vi "2 int to real conversion.vi"(9 "reale in":dbl format="%.20g", 10 "MW 15 0 in":i32=7537, 11 "MW 31 16 in":i32=17309) -> (0 "MW 15 0 out":i16=7537, 1 "MW 31 16 out":i16=17309, 2 "reale out":dbl format="%.20g")   [LabVIEW 2019]
panel:
  out "Boolean array":bool[](array[boolean])
  out "exponent":dbl
  out "mantissa":dbl
  out "appended array 2":bool[](array[boolean])
  out "appended array":bool[](array[boolean])
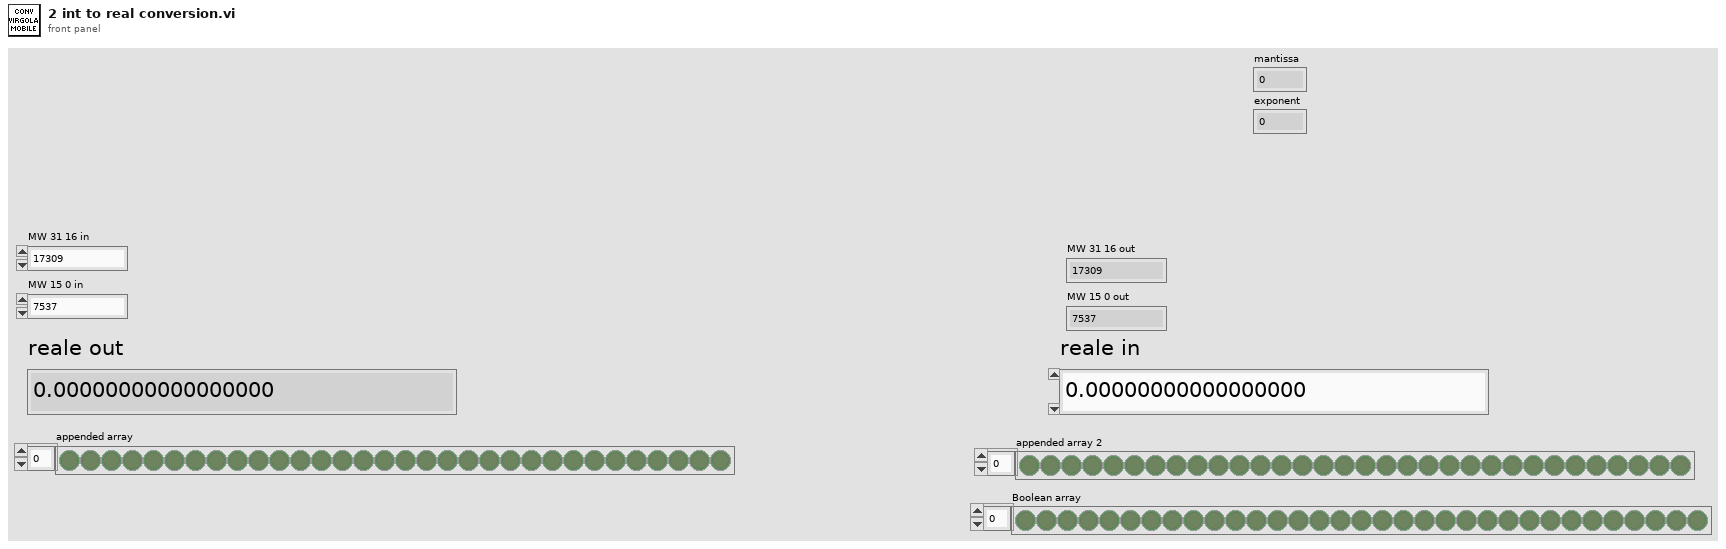
[diagram p1: front panel]
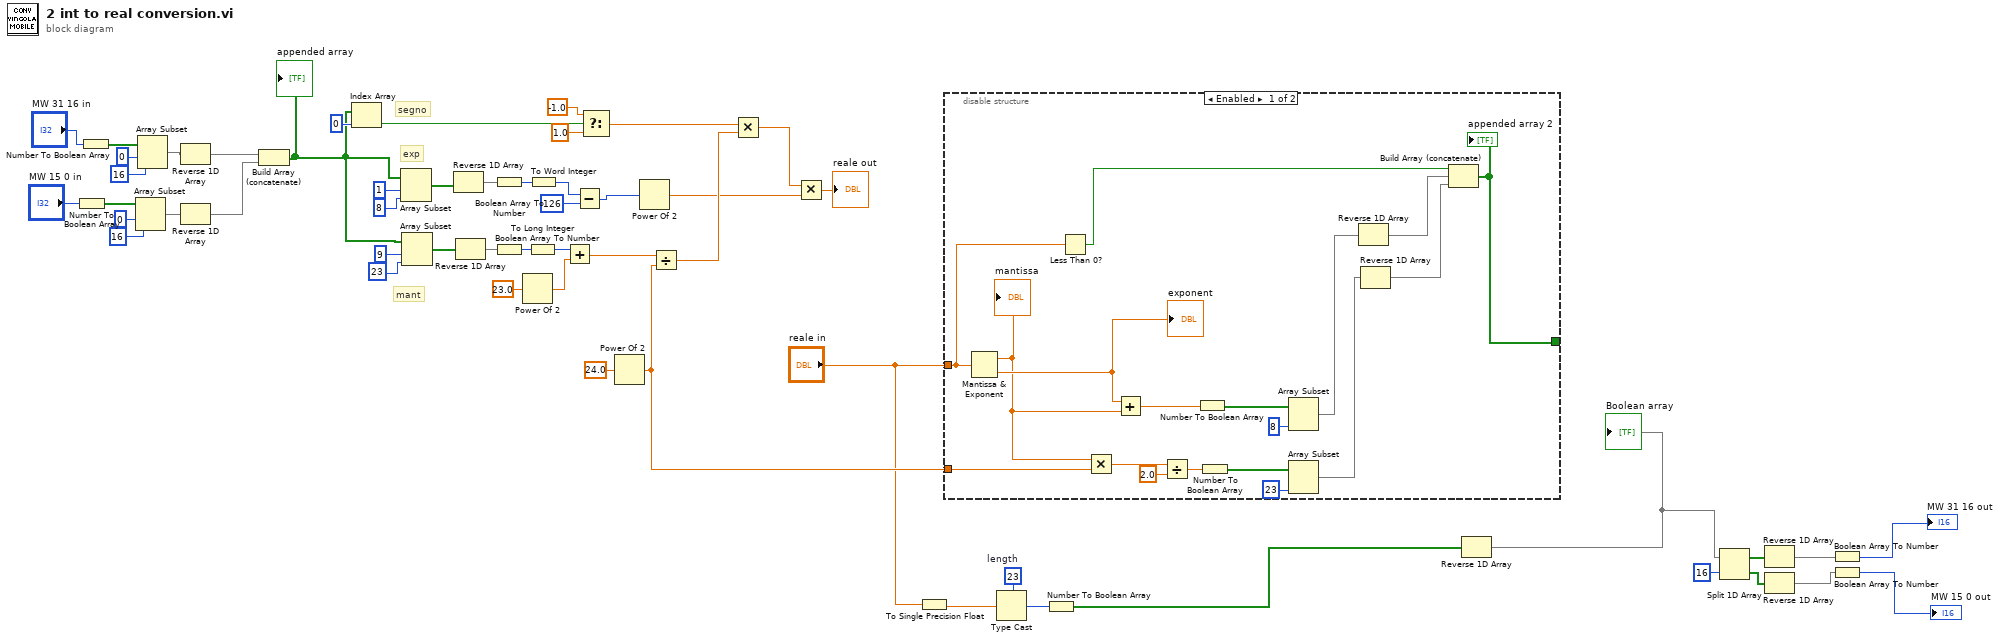
[diagram p0: block diagram]
diagram:
  w8 = 23  # length
  # "mant"
  # "segno"
  # "exp"
  n1 = Number To Boolean Array(number="MW 15 0 in") -> (Boolean array=w54:bool[])
  n2 = Number To Boolean Array(number="MW 31 16 in") -> (Boolean array=w49:bool[])
  n3 = Array Subset(array=w54, index=0, length=16) -> (w35:bool[])
  n4 = Array Subset(array=w49, index=0, length=16) -> (w37:bool[])
  n5 = Reverse 1D Array(array=w37) -> (reversed array=w36:bool[])
  n6 = Reverse 1D Array(array=w35) -> (reversed array=w29:bool[])
  n7 = Build Array (concatenate)(w36, w29) -> (w38:bool[])
  "appended array" <- w38
  n8 = Index Array(array=w38, index=0) -> (element=w33:bool)
  n9 = Array Subset(array=w38, index=1, length=8) -> (w17:bool[])
  n10 = Array Subset(array=w38, index=9, length=23) -> (w18:bool[])
  n11 = Reverse 1D Array(array=w17) -> (reversed array=w16:bool[])
  n12 = Reverse 1D Array(array=w18) -> (reversed array=w15:bool[])
  n13 = Boolean Array To Number(Boolean array=w16) -> (number=w28:u32)
  n14 = Boolean Array To Number(Boolean array=w15) -> (number=w25:u32)
  n15 = Power Of 2(x=23.0) -> (2^x=w12:dbl)
  n16 = To Long Integer(number=w25) -> (32bit integer=w24:i32)
  n17 = To Word Integer(number=w28) -> (16bit integer=w27:i16)
  n18 = Add(x=w24, y=w12) -> (x+y=w39:dbl)
  n19 = Subtract(x=w27, y=i16 126) -> (x-y=w21:i16)
  n20 = Select(t=-1.0 ("y"), s=w33, f=1.0) -> (s? t:f=w32:dbl)
  n21 = Power Of 2(x=24.0) -> (2^x=w11:dbl)
  n22 = Power Of 2(x=w21) -> (2^x=w22:dbl)
  n23 = Divide(x=w39, y=w11) -> (x/y=w23:dbl)
  n24 = Multiply(x=w32, y=w23) -> (x*y=w34:dbl)
  n25 = Multiply(x=w34, y=w22) -> (x*y=→"reale out":dbl)
  n26 = To Single Precision Float(number="reale in") -> (single precision float=w9:sgl)
  n27 = disable-structure shown="Enabled" {
    disable-tunnel: w11 -> [w59 _]
    disable-tunnel: "reale in" -> [w56 _]
    disable-tunnel: [w55 _] -> _
    frame Enabled {
      n28 = Mantissa & Exponent(0:w56) -> (1:w57:dbl, 2:w58:dbl)
      "mantissa" <- w57
      "exponent" <- w58
      n29 = Less Than 0?(x=w56) -> (x < 0?=w71:bool)
      n30 = Multiply(x=w57, y=w59) -> (x*y=w64:dbl)
      n31 = Add(x=w58, y=w57) -> (x+y=w69:dbl)
      n32 = Divide(x=w64, y=2.0) -> (x/y=w65:dbl)
      n33 = Number To Boolean Array(number=w69) -> (Boolean array=w70:bool[])
      n34 = Number To Boolean Array(number=w65) -> (Boolean array=w67:bool[])
      n35 = Array Subset(array=w70, length=8) -> (w63:bool[])  [unwired: 1 in]
      n36 = Array Subset(array=w67, length=23) -> (w62:bool[])  [unwired: 1 in]
      n37 = Reverse 1D Array(array=w63) -> (reversed array=w61:bool[])
      n38 = Reverse 1D Array(array=w62) -> (reversed array=w60:bool[])
      n39 = Build Array (concatenate)(w71, w61, w60) -> (w55:bool[])
      "appended array 2" <- w55
    }
    frame Disabled {
    }
  }
  n40 = Type Cast(type=w8, x=w9) -> (*(type *) &x=w7:i32)
  n41 = Number To Boolean Array(number=w7) -> (Boolean array=w6:bool[])
  n42 = Reverse 1D Array(array=w6) -> (reversed array=w1:bool[])
  "Boolean array" <- w1
  n43 = Split 1D Array(array=w1, index=16) -> (first subarray=w14:bool[], second subarray=w13:bool[])
  n44 = Reverse 1D Array(array=w14) -> (reversed array=w3:bool[])
  n45 = Reverse 1D Array(array=w13) -> (reversed array=w2:bool[])
  n46 = Boolean Array To Number(Boolean array=w3) -> (number=→"MW 31 16 out":u32)
  n47 = Boolean Array To Number(Boolean array=w2) -> (number=→"MW 15 0 out":u32)
